vi "Teleop_System_Acquire_Decide.vi"(11 "Teleop Elapsed Seconds":dbl) -> ()   [LabVIEW 2019]
uses:
  <vilib>/Rock Robotics/WPI/Joystick/XBox Axes Indexer.ctl
  <vilib>/Rock Robotics/WPI/Joystick/XBox Buttons Indexer.ctl
  <vilib>/Rock Robotics/WPI/ThirdParty/JAS_Junk/TrajLib/Conv_POSE2D_SI_Eng.vi
  <vilib>/Rock Robotics/WPI/ThirdParty/JAS_Junk/TrajLib/VI/Util_GetTime_U32.vi
  <vilib>/Rock Robotics/WPI/ThirdParty/JAS_Junk/TrajLib/VI/numCmd_Send_Generic.vi
  <vilib>/Rock Robotics/WPI/ThirdParty/JAS_Junk/TrajLib/Conv_Meters_Feet.vi
  <vilib>/Rock Robotics/WPI/ThirdParty/JAS_Junk/TrajLib/Conv_Radians_Deg.vi
  <vilib>/Rock Robotics/WPI/ThirdParty/JAS_Junk/TrajLib/VI/numCmd_ObtainQueue_Generic.vi
  <vilib>/Rock Robotics/WPI/ThirdParty/JAS_Junk/TrajLib/VI/Util_GetTime_U64.vi
  Swerve_Drive_System/SWERVE_DRIVE_GLOBALS.vi
  <vilib>/Rock Robotics/WPI/Utilities/WPI_GetSetVariantRefNum.vi
  <vilib>/Rock Robotics/Network Tables/NT Write Numeric Array.vi
  <vilib>/Rock Robotics/Network Tables/NT Write Boolean Array.vi
  Sweve_Trajectory_Following/SWERVE_TRAJECTORY_GLOBALS.vi
  <vilib>/Rock Robotics/WPI/ThirdParty/JAS_Junk/TrajLib/Trajectory_Library.lvlib
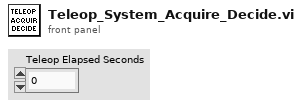
[diagram p1: front panel]
types:
  T1 = typedef "XBox Axes Indexer.ctl" = enum16{"Left X", "Left Y", "Left Trigger", "Right Trigger", "Right X", "Right Y"}
  T2 = typedef "XBox Buttons Indexer.ctl" = enum16{"A", "B", "X", "Y", "Left Bumper", "Right Bumper", "Back", "Start", "Left Joystick", "Right Joystick"}
  T3 = typedef "WPI_JoystickDevRef.ctl" = cluster{"Device":T4}
  T4 = typedef "WPI_JoystickDeviceEnum.ctl" = enum16{"USB 0", "USB 1", "USB 2", "USB 3", "USB 4", "USB 5"}
  T5 = typedef "Trajectory_Library.lvlib/CHASSIS_SPEEDS.ctl" = cluster{"vX":dbl, "vY":dbl, "vOmega":dbl}
  T6 = typedef "Trajectory_Library.lvlib/TRAJ_STATE.ctl" = cluster{"TimeSeconds":dbl, "Velocity":dbl, "Acceleration":dbl, "POSE":T7, "Curvature":dbl}
  T7 = typedef "Trajectory_Library.lvlib/POSE2D.ctl" = cluster{"TRANSLATION":T8, "ROTATION":T9}
  T8 = typedef "Trajectory_Library.lvlib/TRANSLATION2D.ctl" = cluster{"X":dbl, "Y":dbl}
  T9 = typedef "Trajectory_Library.lvlib/ROTATION2D.ctl" = cluster{"VALUE":dbl, "COS":dbl, "SIN":dbl}
  T10 = cluster{"Error Pose":T7, "X Corr":dbl, "Y Corr":dbl}
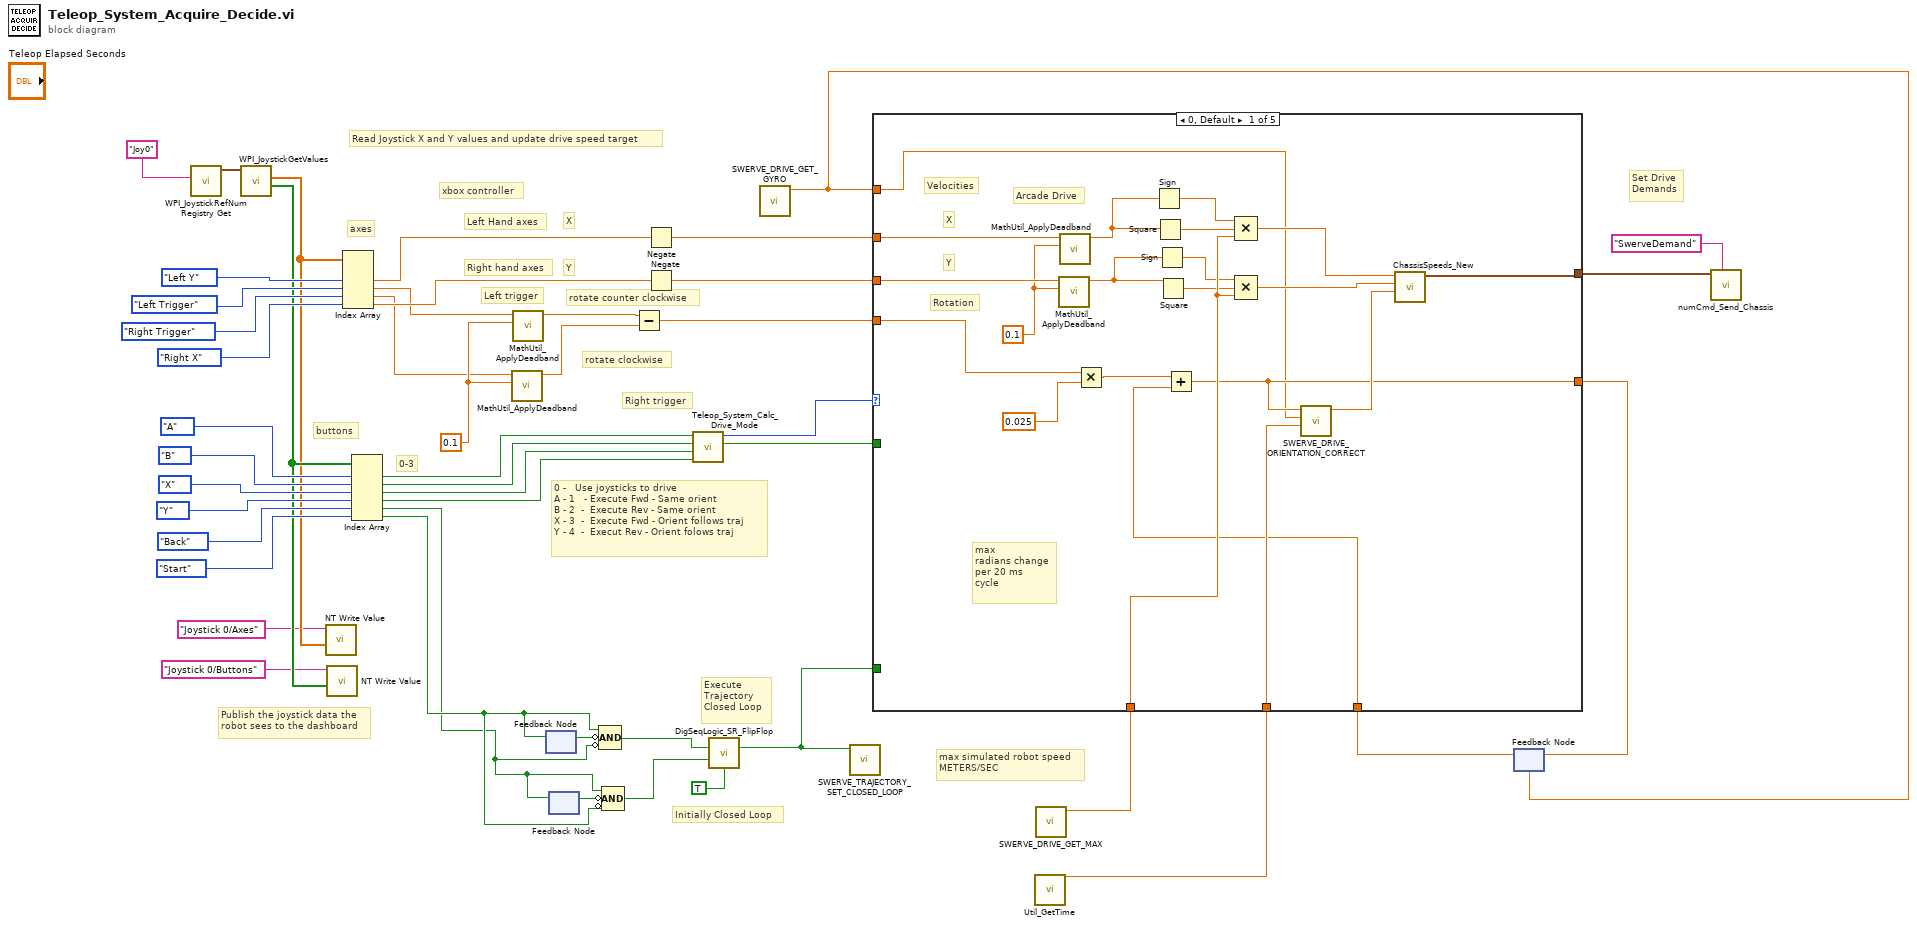
[diagram p0: block diagram]
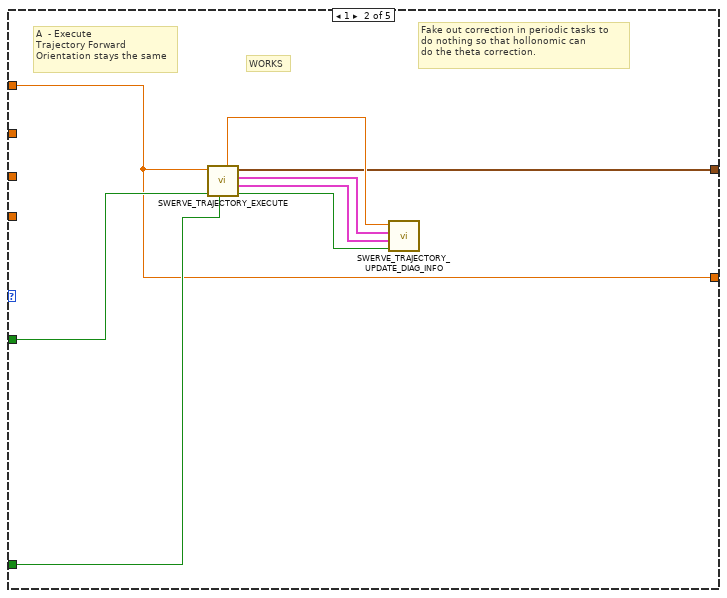
[diagram p2: hidden frame]
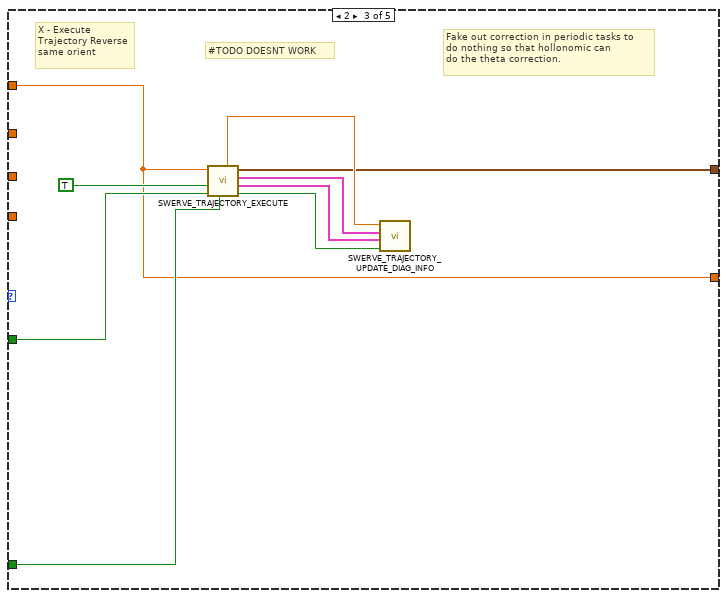
[diagram p3: hidden frame]
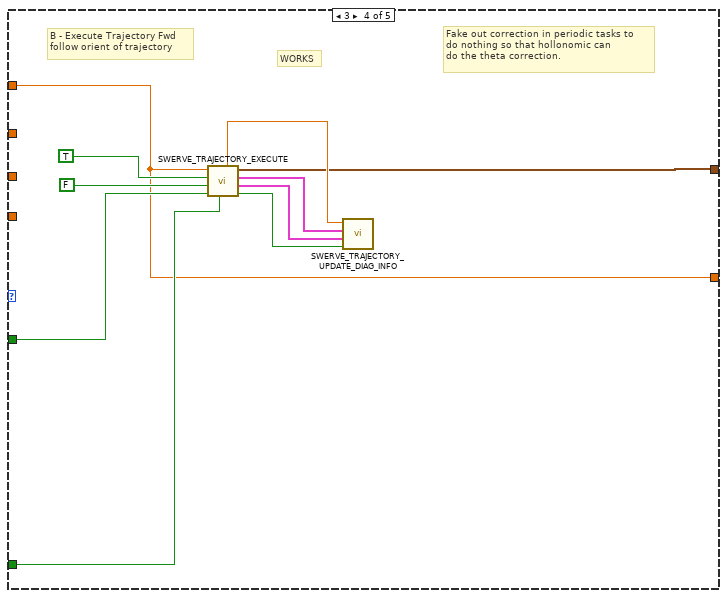
[diagram p4: hidden frame]
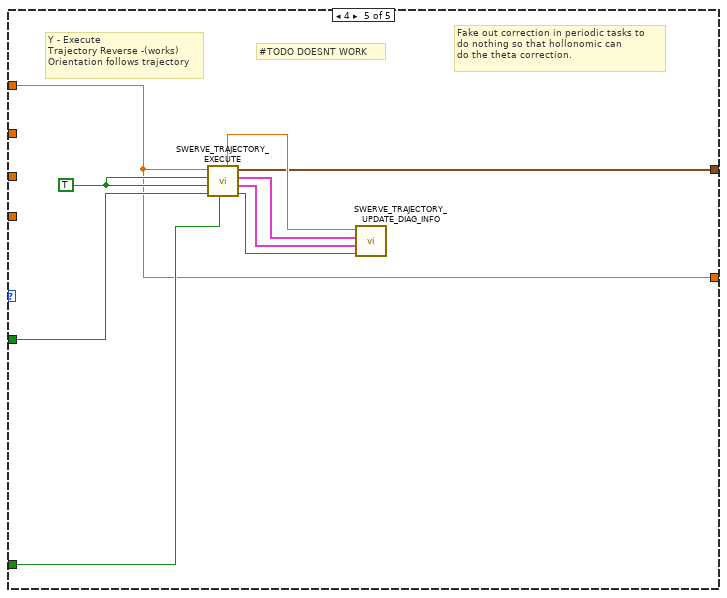
[diagram p5: hidden frame]
diagram:
  w32 = 0.1 ("Deadband")
  # "0 -   Use joysticks to drive\nA - 1   - Execute Fwd - Same orient\nB - 2  -  Execute Rev - Same orient\nX - 3  -  Execute Fwd - Orient follows traj\nY - 4  -  Execut Rev - Orient folows traj"
  # "Execute\nTrajectory\nClosed Loop"
  # "Set Drive\nDemands"
  # "Initially Closed Loop"
  # "0-3"
  # "xbox controller"
  # "Left trigger"
  # "rotate counter clockwise"
  # "Right trigger"
  # "rotate clockwise"
  # "Left Hand axes"
  # "Right hand axes"
  # "Y"
  # "X"
  # "buttons"
  # "axes"
  # "max simulated robot speed\nMETERS/SEC"
  # "Publish the joystick data the\nrobot sees to the dashboard"
  # "Read Joystick X and Y values and update drive speed target"
  n1 = call <vilib>:"WPI_JoystickRefNum Registry Get.vi"("refnum name"="Joy0") -> ("JoystickDevRef"=w12:T3)  [unwired: 1 in, 9 out]
  n2 = call <vilib>:"WPI_JoystickGetValues.vi"("JoystickDevRef"=w12) -> ("Buttons"=w16:bool[], "Axes"=w15:dbl[])  [unwired: 6 in, 3 out]
  n3 = call-poly <vilib>:"NT Write Value.vi"("value"=w15, "name"="Joystick 0/Axes" ("Name")) -> ()  [unwired: 9 in, 1 out]
  n4 = call-poly <vilib>:"NT Write Value.vi"("value"=w16, "name"="Joystick 0/Buttons" ("Name")) -> ()  [unwired: 9 in, 1 out]
  n5 = Index Array(array=w15, index #2=XBox_Axes_Indexer."Left Y" ("XBox Axes"), index #3=XBox_Axes_Indexer."Left Trigger" ("XBox Axes"), index #4=XBox_Axes_Indexer."Right Trigger" ("XBox Axes"), index #5=XBox_Axes_Indexer."Right X" ("XBox Axes")) -> (element #2=w24:dbl, element #3=w6:dbl, element #4=w4:dbl, element #5=w25:dbl)  [unwired: 1 in, 1 out]
  n6 = Index Array(array=w16, index #1=XBox_Buttons_Indexer."A" ("XBox Buttons"), index #2=XBox_Buttons_Indexer."B" ("XBox Buttons"), index #3=XBox_Buttons_Indexer."X" ("XBox Buttons"), index #4=XBox_Buttons_Indexer."Y" ("XBox Buttons"), index #5=XBox_Buttons_Indexer."Back" ("XBox Buttons"), index #6=XBox_Buttons_Indexer."Start" ("XBox Buttons")) -> (element #1=w17:bool, element #2=w26:bool, element #3=w27:bool, element #4=w43:bool, element #5=w30:bool, element #6=w31:bool)
  n7 = call <vilib>:"MathUtil_ApplyDeadband.vi"("Deadband"=w32, "Value"=w4) -> ("Result"=w3:dbl)  [unwired: 9 in]
  n8 = call <vilib>:"MathUtil_ApplyDeadband.vi"("Deadband"=w32, "Value"=w6) -> ("Result"=w5:dbl)  [unwired: 9 in]
  n9 = feedback #1() -> (w28:bool)  [unwired: 1 in]
  n10 = feedback-in #1(w31) -> ()
  n11 = feedback #2() -> (w29:bool)  [unwired: 1 in]
  n12 = feedback-in #2(w30) -> ()
  n13 = Compound Arithmetic op=AND(w31, invert w28, invert w30) -> (w34:bool)
  n14 = Compound Arithmetic op=AND(w30, invert w29, invert w31) -> (w35:bool)
  n15 = Subtract(x=w5, y=w3) -> (x-y=w21:dbl)
  n16 = Negate(x=w24) -> (-x=w22:dbl)
  n17 = Negate(x=w25) -> (-x=w23:dbl)
  n18 = call "Teleop_System_Calc_Drive_Mode.vi"("Traj Rev Follow Orient"=w43, "Traj Rev Same Orient"=w27, "Traj Fwd Follow Orient"=w26, "Traj Fwd Same Orient"=w17) -> ("Dirve Mode Changed"=w19:bool, "Drive Mode"=w18:i32)  [unwired: 6 in]
  n19 = call <vilib>:"DigSeqLogic_SR_FlipFlop.vi"("Set"=w34, "Reset"=w35, "Initial Value"=TRUE) -> ("Output"=w36:bool)  [unwired: 11 in, 1 out]
  n20 = call "SWERVE_DRIVE_GET_GYRO.vi"() -> ("Gyro Heading Radians"=w8:dbl)  [unwired: 11 in]
  n21 = call "SWERVE_TRAJECTORY_SET_CLOSED_LOOP.vi"("AUTO_CLOSED_LOOP"=w36) -> ()  [unwired: 11 in]
  n22 = call <vilib>:"Util_GetTime.vi"() -> ("FPGA_Time_Seconds"=w10:dbl)  [unwired: 9 in, 2 out]
  n23 = call "SWERVE_DRIVE_GET_MAX.vi"() -> ("Max Wheel Vel (Meter/Sec)"=w20:dbl)  [unwired: 10 in, 1 out]
  n24 = feedback #3(w8) -> (w7:dbl)
  n25 = case shown="0, Default" w18 {
    tunnel: w23 -> [w57 _ _ _ _]
    tunnel: w20 -> [w68 _ _ _ _]
    tunnel: w19 -> [_ w76 w85 w95 w104]
    tunnel: w22 -> [w59 _ _ _ _]
    tunnel: w21 -> [w61 _ _ _ _]
    tunnel: w8 -> [w49 w69 w77 w86 w96]
    tunnel: w36 -> [_ w75 w83 w92 w102]
    tunnel: [w53 w70 w78 w87 w97] -> w2
    tunnel: w10 -> [w52 _ _ _ _]
    tunnel: [w50 w69 w77 w86 w96] -> w9
    tunnel: w7 -> [w48 _ _ _ _]
    frame 0, Default {
      w56 = 0.1 ("Deadband")
      # "Velocities"
      # "Rotation"
      # "max \nradians change\nper 20 ms\ncycle"
      # "Y"
      # "X"
      # "Arcade Drive"
      n26 = call <vilib>:"MathUtil_ApplyDeadband.vi"("Deadband"=w56, "Value"=w57) -> ("Result"=w60:dbl)  [unwired: 9 in]
      n27 = call <vilib>:"MathUtil_ApplyDeadband.vi"("Deadband"=w56, "Value"=w59) -> ("Result"=w58:dbl)  [unwired: 9 in]
      n28 = Multiply(x=w61, y=0.025) -> (x*y=w63:dbl)
      n29 = Sign(1:w58) -> (0:w66:dbl)
      n30 = Square(x=w58) -> (x^2=w67:dbl)
      n31 = Sign(1:w60) -> (0:w64:dbl)
      n32 = Square(x=w60) -> (x^2=w65:dbl)
      n33 = Add(x=w63, y=w48) -> (x+y=w50:dbl)
      n34 = Compound Arithmetic op=MULTIPLY(w66, w67, w68) -> (w55:dbl)
      n35 = Compound Arithmetic op=MULTIPLY(w64, w65, w68) -> (w54:dbl)
      n36 = call "SWERVE_DRIVE_ORIENTATION_CORRECT.vi"("FPGA_Time_Seconds"=w52, "Gyro Heading Radians"=w49, "Drv Rotation Orentation Dmd  Radians"=w50) -> ("CO-ControlOutput"=w51:dbl)  [unwired: 8 in]
      n37 = call <vilib>:"ChassisSpeeds_New.vi"("vAngular"=w51, "vY"=w54, "vX"=w55) -> ("CHASSIS"=w53:T5)  [unwired: 8 in]
    }
    frame 1 {
      # "Fake out correction in periodic tasks to \ndo nothing so that hollonomic can\ndo the theta correction."
      # "WORKS"
      # "A  - Execute\nTrajectory Forward\nOrientation stays the same"
      n38 = call "SWERVE_TRAJECTORY_EXECUTE.vi"("EnableClosedLoop"=w75, "Init"=w76, "Gyro Heading\nRAD"=w69) -> ("AtReference"=w71:bool, "OutputTRAJ_STATE"=w72:T6, "Error and Corr"=w73:T10, "Chassis Velocity Target"=w70:T5, "Orientation Target"=w74:dbl)  [unwired: 4 in]
      n39 = call "SWERVE_TRAJECTORY_UPDATE_DIAG_INFO.vi"("AtReference"=w71, "OutputTRAJ_STATE"=w72, "Error and Corr"=w73, "Orientation Target"=w74) -> ()  [unwired: 8 in]
    }
    frame 2 {
      # "Fake out correction in periodic tasks to \ndo nothing so that hollonomic can\ndo the theta correction."
      # "#TODO DOESNT WORK"
      # "X - Execute \nTrajectory Reverse\nsame orient"
      n40 = call "SWERVE_TRAJECTORY_EXECUTE.vi"("EnableClosedLoop"=w83, "Init"=w85, "Reverse"=TRUE, "Gyro Heading\nRAD"=w77) -> ("AtReference"=w79:bool, "OutputTRAJ_STATE"=w80:T6, "Error and Corr"=w81:T10, "Chassis Velocity Target"=w78:T5, "Orientation Target"=w82:dbl)  [unwired: 3 in]
      n41 = call "SWERVE_TRAJECTORY_UPDATE_DIAG_INFO.vi"("AtReference"=w79, "OutputTRAJ_STATE"=w80, "Error and Corr"=w81, "Orientation Target"=w82) -> ()  [unwired: 8 in]
    }
    frame 3 {
      # "Fake out correction in periodic tasks to \ndo nothing so that hollonomic can\ndo the theta correction."
      # "WORKS"
      # "B - Execute Trajectory Fwd \nfollow orient of trajectory"
      n42 = call "SWERVE_TRAJECTORY_EXECUTE.vi"("EnableClosedLoop"=w92, "Init"=w95, "Reverse"=FALSE, "Follow Orientation"=TRUE ("Reverse"), "Gyro Heading\nRAD"=w86) -> ("AtReference"=w88:bool, "OutputTRAJ_STATE"=w89:T6, "Error and Corr"=w90:T10, "Chassis Velocity Target"=w87:T5, "Orientation Target"=w91:dbl)  [unwired: 2 in]
      n43 = call "SWERVE_TRAJECTORY_UPDATE_DIAG_INFO.vi"("AtReference"=w88, "OutputTRAJ_STATE"=w89, "Error and Corr"=w90, "Orientation Target"=w91) -> ()  [unwired: 8 in]
    }
    frame 4 {
      w103 = TRUE ("Reverse")
      # "Fake out correction in periodic tasks to \ndo nothing so that hollonomic can\ndo the theta correction."
      # "#TODO DOESNT WORK"
      # "Y - Execute\nTrajectory Reverse -(works)\nOrientation follows trajectory"
      n44 = call "SWERVE_TRAJECTORY_EXECUTE.vi"("EnableClosedLoop"=w102, "Init"=w104, "Reverse"=w103, "Follow Orientation"=w103, "Gyro Heading\nRAD"=w96) -> ("AtReference"=w98:bool, "OutputTRAJ_STATE"=w99:T6, "Error and Corr"=w100:T10, "Chassis Velocity Target"=w97:T5, "Orientation Target"=w101:dbl)  [unwired: 2 in]
      n45 = call "SWERVE_TRAJECTORY_UPDATE_DIAG_INFO.vi"("AtReference"=w98, "OutputTRAJ_STATE"=w99, "Error and Corr"=w100, "Orientation Target"=w101) -> ()  [unwired: 8 in]
    }
  }
  n46 = feedback-in #3(w9) -> ()
  n47 = call <vilib>:"numCmd_Send_Chassis.vi"("Command Name"="SwerveDemand", "Chassis Speeds"=w2) -> ()  [unwired: 9 in, 1 out]
